vi "Uniform White Noise.vi"(7 "initialize?":bool=TRUE, 9 "seed":i32=-1, 10 "amplitude":dbl=1.0 format="%0.2f", 11 "samples":i32=128) -> (0 "error":i32, 3 "uniform white noise":dbl[](array[numeric]))   [LabVIEW 2014, in "NI_AALBase.lvlib"]
doc: "Generates a uniformly distributed, pseudorandom pattern whose values are in the range [-a:a], where a is the absolute value of <B>amplitude</B>."
uses:
  NI_AALBase.lvlib
  lvanlys.dll
panel:
  # "Uniform White Noise"
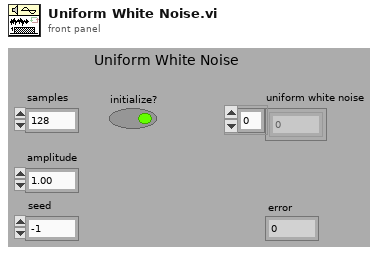
[diagram p1: front panel]
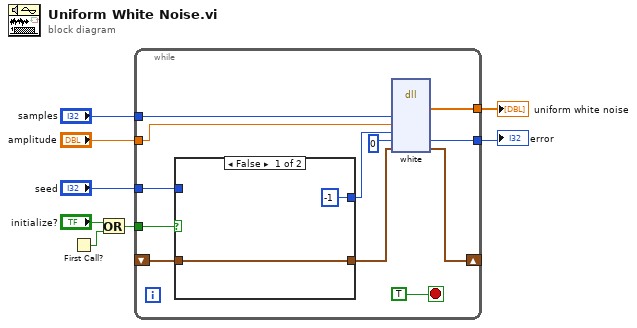
[diagram p0: block diagram]
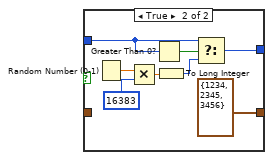
[diagram p2: hidden frame]
diagram:
  n1 = First Call?() -> (First Call?: T/F=w3:bool)
  n2 = Or(x="initialize?", y=w3) -> (x .or. y?=w4:bool)
  n3 = while {
    tunnel: [w20] -> w8
    tunnel: "seed" -> [w14]
    tunnel: "amplitude" -> [w19]
    tunnel: "samples" -> [w18]
    shift-right: [w16] -> _
    shift-left: _ -> [w12]
    tunnel: w4 -> [w13]
    tunnel: [w9] -> w1
    stop <- TRUE stop-if-true
    n4 = case shown="False" w13 {
      tunnel: w12 -> [w22 _]
      tunnel: [w22 cluster{"xSeed":i32, "ySeed":i32, "zSeed":i32} {"xSeed"=1234, "ySeed"=2345, "zSeed"=3456} ("RNGState")] -> w11
      tunnel: [-1 ("seed") w28] -> w10
      tunnel: w14 -> [_ w29]
      frame False {
      }
      frame True {
        n5 = Random Number (0-1)() -> (number: 0 to 1=w26:dbl)
        n6 = Multiply(x=w26, y=16383 ("x")) -> (x*y=w27:dbl)
        n7 = Greater Than 0?(x=w29) -> (x > 0?=w30:bool)
        n8 = To Long Integer(number=w27) -> (32bit integer=w25:i32)
        n9 = Select(t=w29, s=w30, f=w25) -> (s? t:f=w28:i32)
      }
    }
    n10 = dll-call lib="C:/Program Files (x86)/National Instruments/LabVIEW 2014/resource/lvanlys.*" fn="white"("size"=w18, "ampl"=w19, "theSeed"=w10, "dsperr"=0, "rng_state"=w11) -> ("xH"=w9:dbl[], "dsperr"=w20:i32, "rng_state"=w16:cluster{"xSeed":i32, "ySeed":i32, "zSeed":i32})  [unwired: 6 in, 4 out]
  }
  "error" <- w8
  "uniform white noise" <- w1
